vi "Pace pluse  interval Measurement.vi"(0 "ref in":T4, 1 "测试 类型":string(combo)="VREF", 5 "tasks in":T3, 7 "Oscilloscope IO":refnum<visa-resource-name>="tcpip0::192.168.40.220::instr", 9 "Data in":variant, 11 "error in (no error)":errorcluster) -> (6 "all  data out":T2={"conditions"={"do test?"=TRUE, "test name"="ib trim test", "user test name"="", "temp"=25.0, "spec min 1"=0.0, "spec max 1"=31.0, "spec min 2"=0.0, "spec max 2"=0.0, "spec units"="dec", "type"=enum."absolute", "vin inital"=2.8, "dwell initial"=0.5, "start"=0.0, "stop"=31.0, "step"=1.0, "dwell"=0.2, "bat imp"=0.0, "lead imp"=0.0, "schamber"="a", "gain"=0.0, "spolarity"="t2r", "as"=0.0, "vs"=0.0, "period"=0.0, "pchamber"="a", "ppolarity"="bip\nbip", "aamp"=0.0, "vamp"=0.0, "rchtime"=0.0, "rate"=0.0, "freq"=0.0, "vin end"=0.0, "dwell end"=0.5, "level a"=0.0, "level b"=0.0, "level c"=0.0, "level d"=0.0, "notes"="", "slew time"=25.0, "pw"=0.0, "times"=0.0, "spec min 3"=0.0, "spec max 3"=31.0, "spec min 4"=0.0, "spec max 4"=0.0}, "data out"=[], "result"=[], "TestArrayIndex"=0, "Result Measurement Head"=[]} {"conditions"."spec max 4" format="%^.3e"; "conditions"."spec min 4" format="%^.3e"; "conditions"."spec max 3" format="%^.3e"; "conditions"."spec min 3" format="%^.3e"; "conditions"."times" format="%^.3e"; "conditions"."pw" format="%^.3e"; "conditions"."slew time" format="%.2f"; "conditions"."level a" format="%^.3e"; "conditions"."freq" format="%^.3e"; "conditions"."rate" format="%^.3e"; "conditions"."rchtime" format="%^.3e"; "conditions"."vamp" format="%^.3e"; "conditions"."aamp" format="%^.3e"; "conditions"."period" format="%^.3e"; "conditions"."vs" format="%^.3e"; "conditions"."as" format="%^.3e"; "conditions"."gain" format="%^.3e"; "conditions"."lead imp" format="%^.3e"; "conditions"."bat imp" format="%^.3e"; "conditions"."spec max 2" format="%^.3e"; "conditions"."spec min 2" format="%^.3e"; "conditions"."level d" format="%^.3e"; "conditions"."level c" format="%^.3e"; "conditions"."level b" format="%^.3e"; "conditions"."dwell end" format="%^.3e"; "conditions"."vin end" format="%^.3e"; "conditions"."dwell" format="%^.3e"; "conditions"."step" format="%^.3e"; "conditions"."stop" format="%^.3e"; "conditions"."start" format="%^.3e"; "conditions"."dwell initial" format="%^.3e"; "conditions"."vin inital" format="%^.3e"; "conditions"."spec max 1" format="%^.3e"; "conditions"."spec min 1" format="%^.3e"; "conditions"."temp" format="%.2f"}, 10 "Measurement":string[](array[string]), 15 "Waveform Graph Cal":waveform(dbl)(graph))   [LabVIEW 2016]
uses:
  AET/TypeDef/Pacemaker ASIC Test_Reference.ctl
  AET/TypeDef/Pacemaker ASIC Test_Task.ctl
  AET/TypeDef/Pacemaker ASIC Test_Condition.ctl
  AET/TypeDef/Pacemaker ASIC Test_Register Mark Type.ctl
  Global Variables/Pacemaker ASIC Test_Save_SN Globals.vi
panel:
  out "Save_SN":path
  out "Pass/Fail":bool
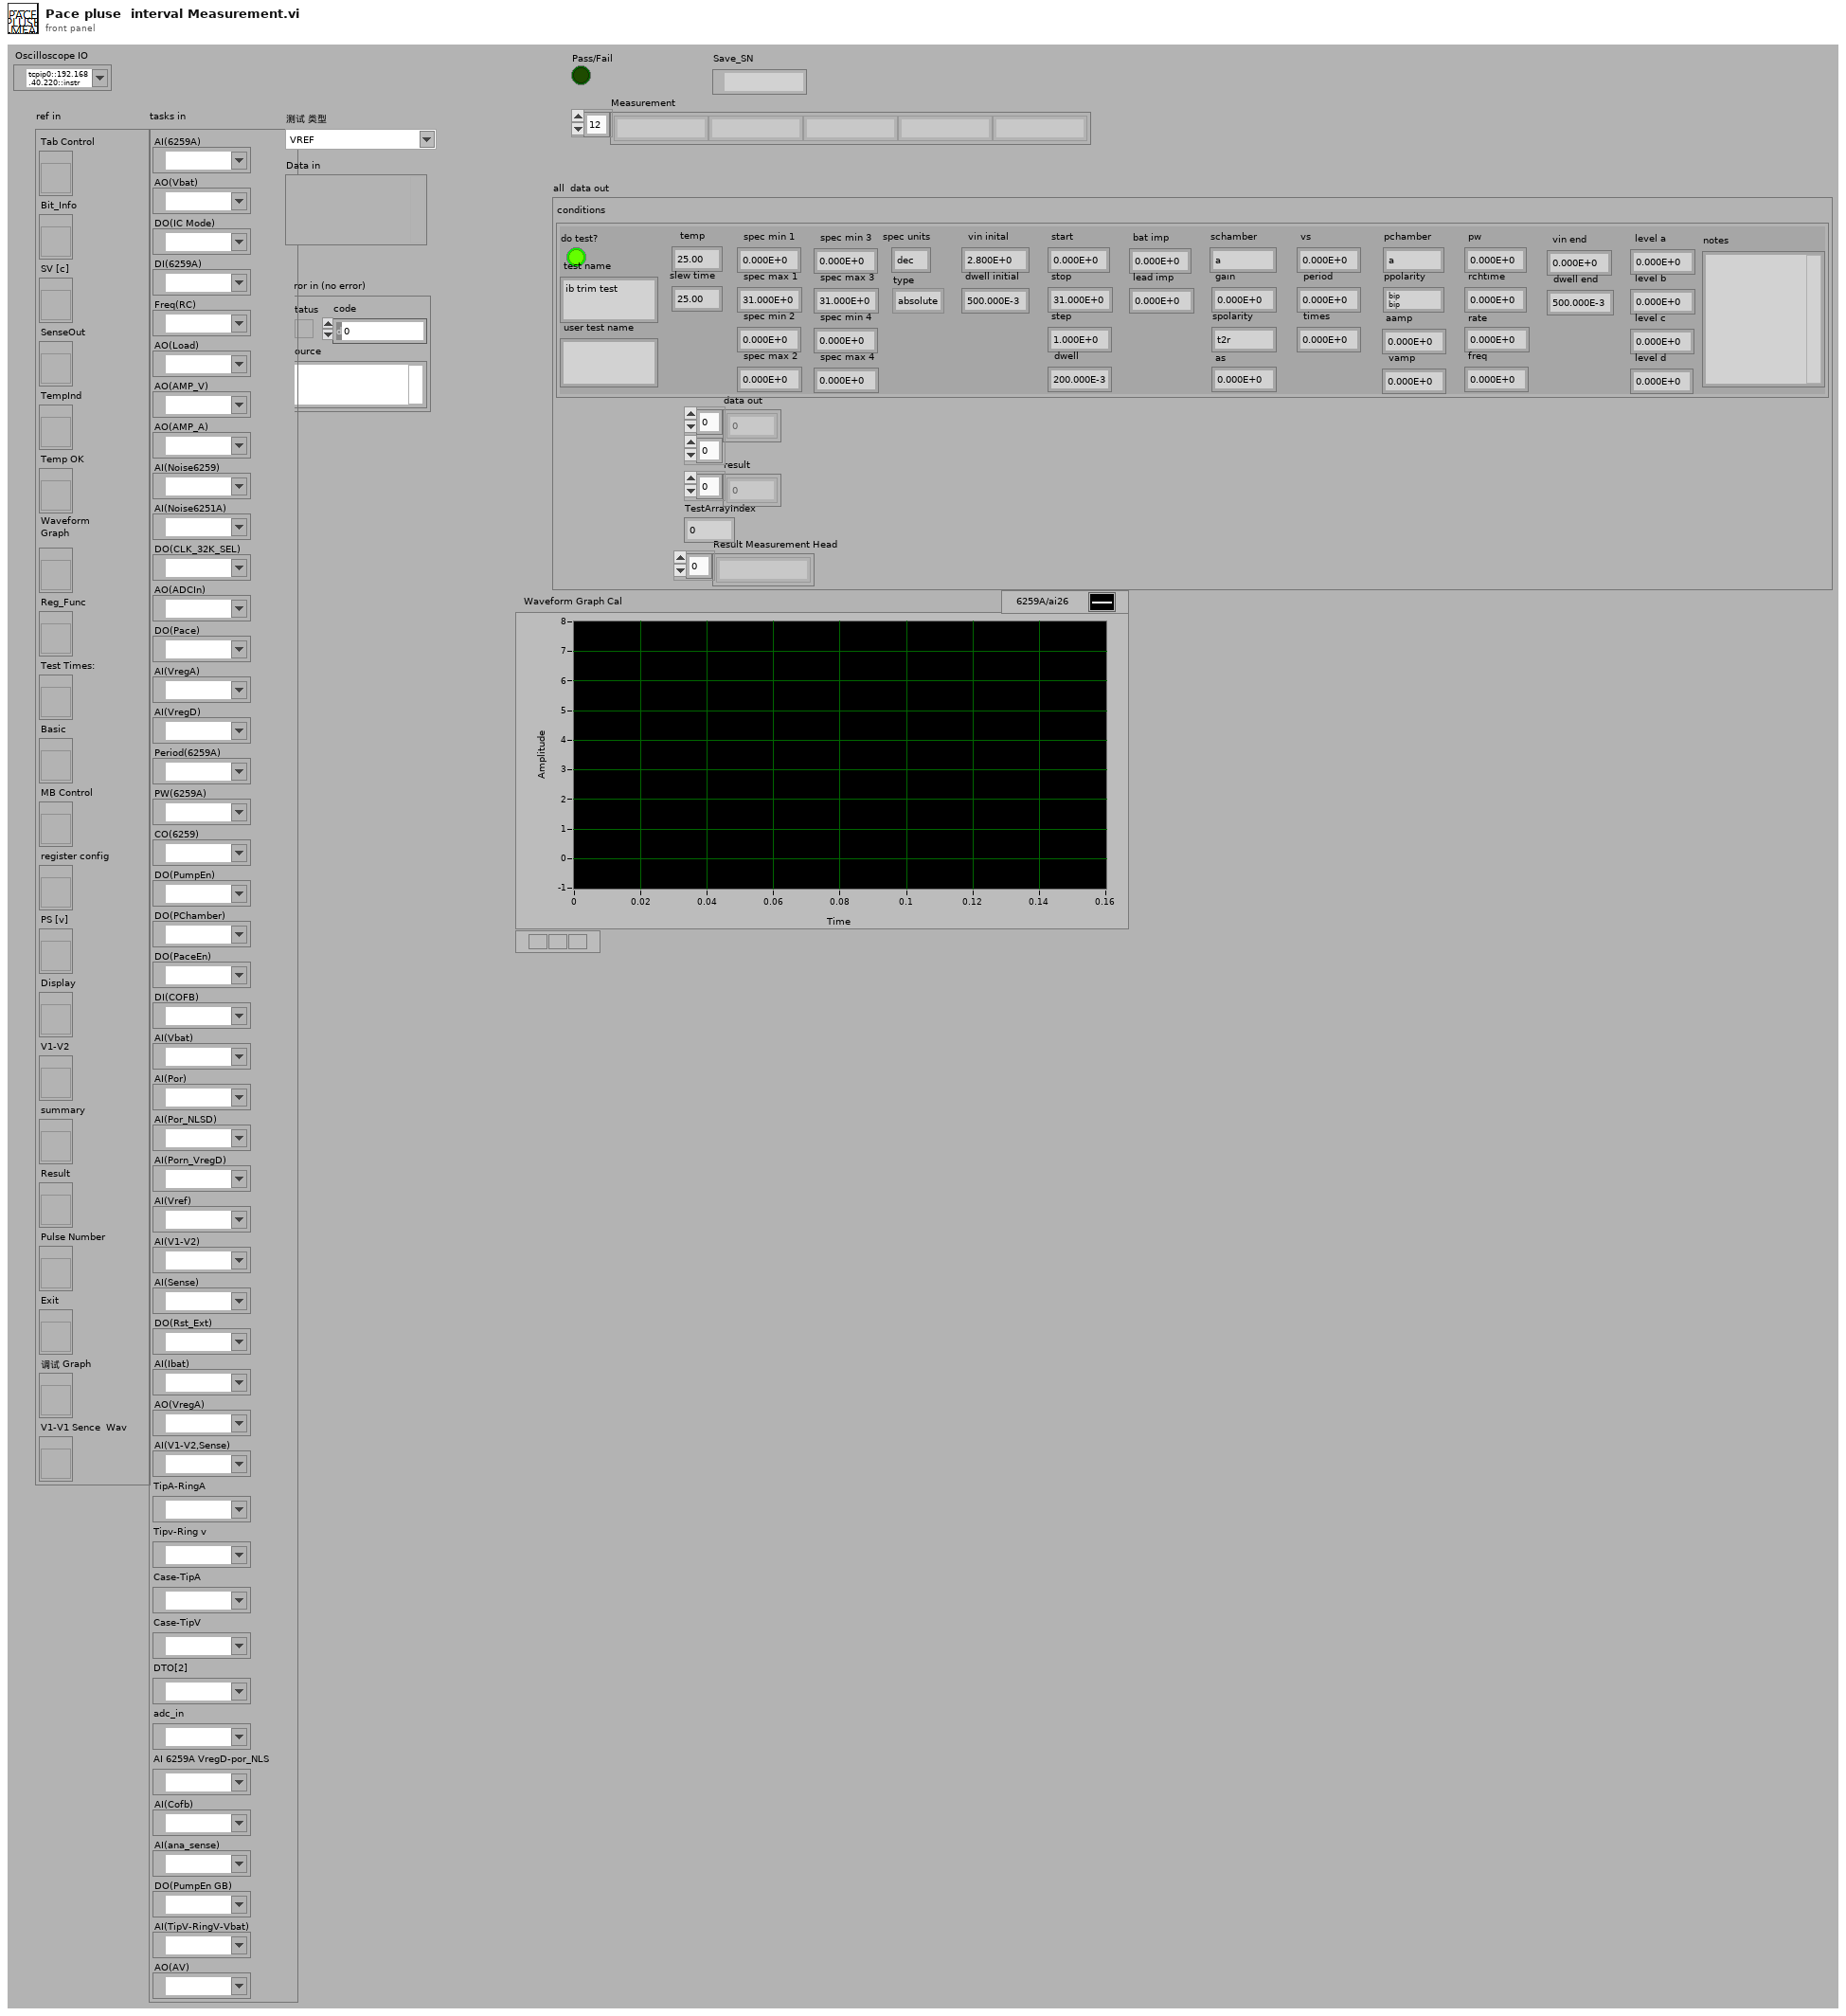
[diagram p1: front panel]
types:
  T1 = typedef "Pacemaker ASIC Test_Condition.ctl" = cluster{"do test?":bool, "test name":string, "user test name":string, "temp":dbl, "spec min 1":dbl, "spec max 1":dbl, "spec min 2":dbl, "spec max 2":dbl, "spec units":string, "type":enum16{"absolute", "v change", "pct change"}, "vin inital":dbl, "dwell initial":dbl, "start":dbl, "stop":dbl, "step":dbl, "dwell":dbl, "bat imp":dbl, "lead imp":dbl, "schamber":string, "gain":dbl, "spolarity":string, "as":dbl, "vs":dbl, "period":dbl, "pchamber":string, "ppolarity":string, "aamp":dbl, "vamp":dbl, "rchtime":dbl, "rate":dbl, "freq":dbl, "vin end":dbl, "dwell end":dbl, "level a":dbl, "level b":dbl, "level c":dbl, "level d":dbl, "notes":string, "slew time":dbl, "pw":dbl, "times":dbl, "spec min 3":dbl, "spec max 3":dbl, "spec min 4":dbl, "spec max 4":dbl}
  T2 = cluster{"conditions":T1, "data out":dbl[][], "result":dbl[], "TestArrayIndex":i32, "Result Measurement Head":string[]}
  T3 = typedef "Pacemaker ASIC Test_Task.ctl" = cluster{"AI(6259A)":refnum<k21>, "AO(Vbat)":refnum<k21>, "DO(IC Mode)":refnum<k21>, "DI(6259A)":refnum<k21>, "Freq(RC)":refnum<k21>, "AO(Load)":refnum<k21>, "AO(AMP_V)":refnum<k21>, "AO(AMP_A)":refnum<k21>, "AI(Noise6259)":refnum<k21>, "AI(Noise6251A)":refnum<k21>, "DO(CLK_32K_SEL)":refnum<k21>, "AO(ADCIn)":refnum<k21>, "DO(Pace)":refnum<k21>, "AI(VregA)":refnum<k21>, "AI(VregD)":refnum<k21>, "Period(6259A)":refnum<k21>, "PW(6259A)":refnum<k21>, "CO(6259)":refnum<k21>, "DO(PumpEn)":refnum<k21>, "DO(PChamber)":refnum<k21>, "DO(PaceEn)":refnum<k21>, "DI(COFB)":refnum<k21>, "AI(Vbat)":refnum<k21>, "AI(Por)":refnum<k21>, "AI(Por_NLSD)":refnum<k21>, "AI(Porn_VregD)":refnum<k21>, "AI(Vref)":refnum<k21>, "AI(V1-V2)":refnum<k21>, "AI(Sense)":refnum<k21>, "DO(Rst_Ext)":refnum<k21>, "AI(Ibat)":refnum<k21>, "AO(VregA)":refnum<k21>, "AI(V1-V2,Sense)":refnum<k21>, " TipA-RingA":refnum<k21>, "Tipv-Ring v":refnum<k21>, " Case-TipA":refnum<k21>, "Case-TipV":refnum<k21>, "DTO[2]":refnum<k21>, "adc_in":refnum<k21>, "AI 6259A VregD-por_NLS":refnum<k21>, "AI(Cofb)":refnum<k21>, "AI(ana_sense)":refnum<k21>, "DO(PumpEn GB)":refnum<k21>, "AI(TipV-RingV-Vbat)":refnum<k21>, "AO(AV)":refnum<k21>}
  T4 = typedef "Pacemaker ASIC Test_Reference.ctl" = cluster{"Tab Control":refnum<vi>, "Bit_Info":refnum<vi>, "SV [c]":refnum<vi>, "SenseOut":refnum<vi>, "TempInd":refnum<vi>, "Temp OK":refnum<vi>, "Waveform \nGraph":refnum<vi>, "Reg_Func":refnum<vi>, "Test Times:":refnum<vi>, "Basic":refnum<vi>, "MB Control":refnum<vi>, "register config":refnum<vi>, "PS [v]":refnum<vi>, "Display":refnum<vi>, "V1-V2":refnum<vi>, "summary":refnum<vi>, "Result":refnum<vi>, "Pulse Number":refnum<vi>, "Exit":refnum<vi>, "调试 Graph":refnum<vi>, "V1-V1 Sence  Wav ":refnum<vi>}
  T5 = typedef "Pacemaker ASIC Test_Register Mark Type.ctl" = enum16{"no action", "TRIM_BANDGAPV", "TRIM_VREGD", "TRIM_VREGA", "TRIM_IBIAS", "TRIM_HPFBW", "TRIM_LPFBW", "TRIM_RC32k", "TRIM_RC1p6k", "TRIM_IBIPT_A", "TRIM_IBIPT_V", "ASGN", "AS", "AUR_UT", "APAMP", "APW", "APUMPGN", "ARCHG", "ABILUNISEL", "VSGN", "VS", "VUR_UT", "VPAMP", "VPW", "VPUMPGN", "VRCHG", "VBILUNISEL", "Test_sel_a", "Test_sel_b", "DTO_SEL", "FBCMEN", "CPEN", "RC1p6kEN", "AntDTM", "ANTENN", "EGMFS REQ", "RC32kEN", "CPUOK", "ENOBLP1", "ENOBLP2", "OBLANK", "PDSA1", "PDSV1", "CSAEN", "CSVEN", "BIR RL", "BIR RH", "MREQ", "RK_SEL", "MRESULT1", "MRESULT2", "TrimOTA_0S1", "TrimOTA_0S2", "TrimOTV_0S1", "TrimOTV_0S2", "ENCASES", "TRIM_HPFBW_H_A", "TRIM_HPFBW_L_A", "TRIM_LPFBW_A", "TRIM_HPFBW_H_V", "TRIM_HPFBW_L_V", "TRIM_LPFBW_V", "R_C_Sel", "PDCHG", "ASIC VVI"}
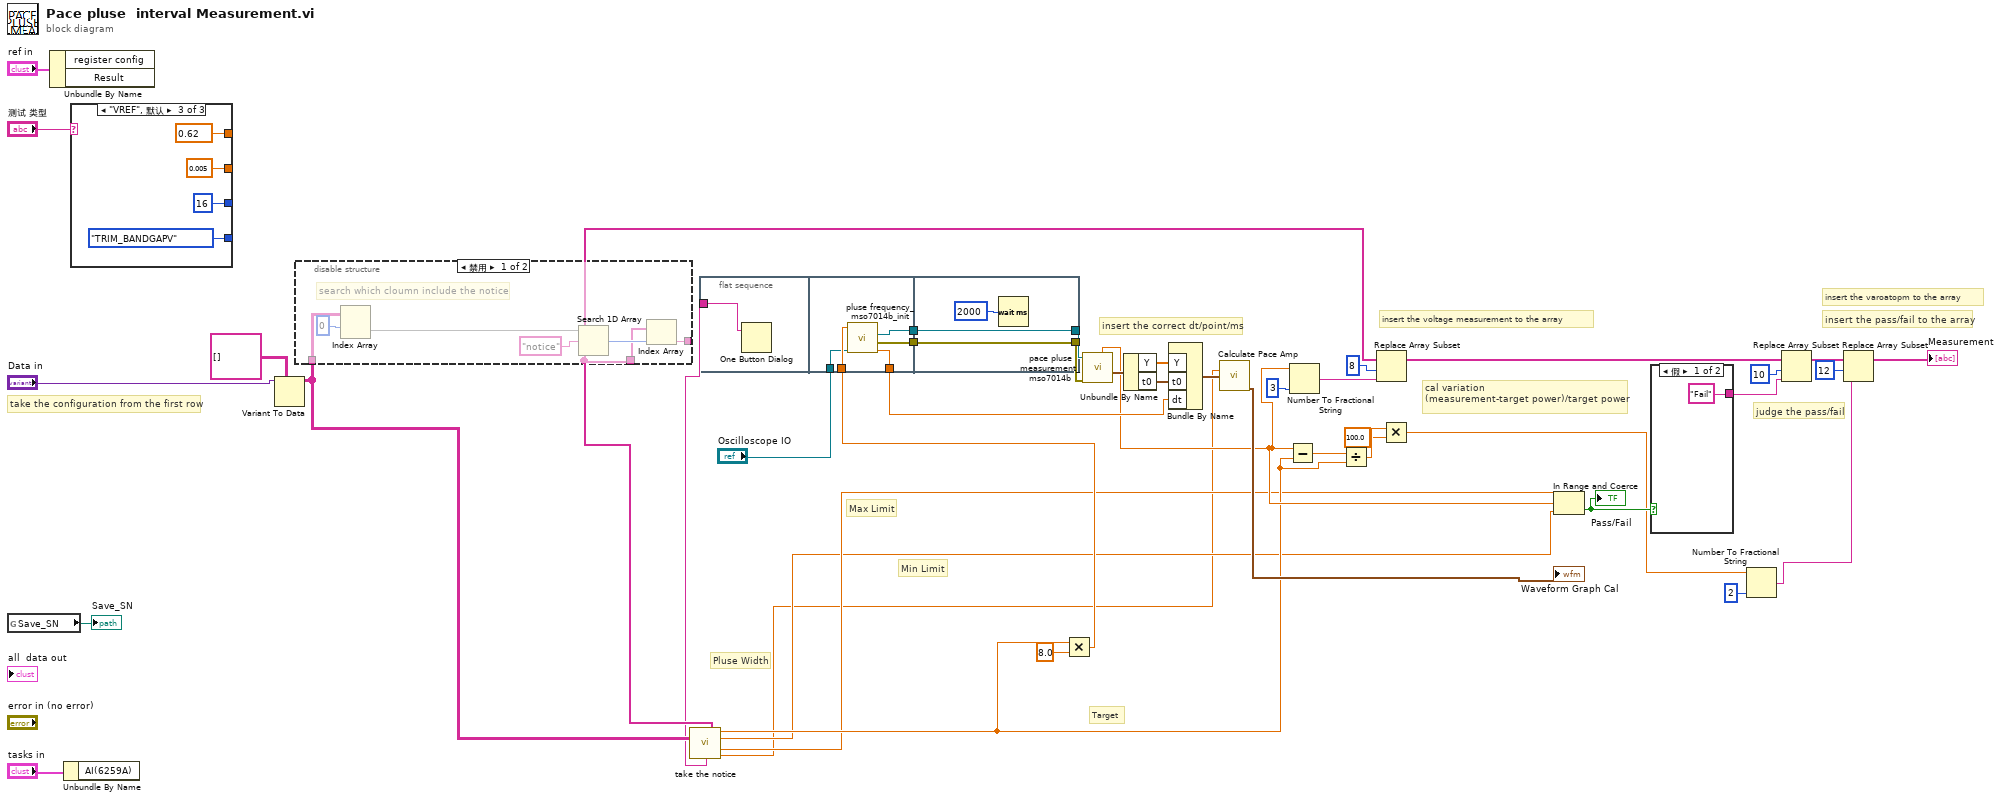
[diagram p0: block diagram]
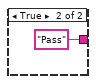
[diagram p3: hidden frame]
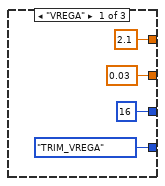
[diagram p4: hidden frame]
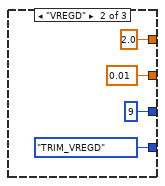
[diagram p5: hidden frame]
diagram:
  # "Pluse Width"
  # "insert the correct dt/point/ms"
  # "take the configuration from the first row"
  # "insert the pass/fail to the array"
  # "insert the varoatopm to the array"
  # "insert the voltage measurement to the array"
  # "judge the pass/fail"
  # "cal variation\n(measurement-target power)/target power"
  # "Target"
  # "Min Limit"
  # "Max Limit"
  n1 = global read "Pacemaker ASIC Test_Save_SN Globals.vi" "Save_SN"() -> (→"Save_SN":path)
  n2 = Unbundle By Name("ref in") -> ()  [unwired: 2 out]
  n3 = Unbundle By Name("tasks in") -> ()  [unwired: 1 out]
  n4 = case shown="\"VREF\", 默认" "测试 类型" {
    tunnel: [Pacemaker_ASIC_Test_Register_Mark_Type."TRIM_VREGA" ("Reg Mark") Pacemaker_ASIC_Test_Register_Mark_Type."TRIM_VREGD" ("Reg Mark") Pacemaker_ASIC_Test_Register_Mark_Type."TRIM_BANDGAPV" ("Reg Mark")] -> _
    tunnel: [2.1 ("y") 2.0 ("y") 0.62 ("y")] -> _
    tunnel: [u8 16 ("y") u8 9 ("y") u8 16 ("y")] -> _
    tunnel: [0.03 ("y") 0.01 ("y") 0.005 ("y")] -> _
    frame "VREGA" {
    }
    frame "VREGD" {
    }
    frame "VREF", Default {
    }
  }
  n5 = Variant To Data(type=string[][] [], Variant="Data in") -> (data=w8:string[][])  [unwired: 1 in, 1 out]
  n6 = call "take the notice.vi"("数组"=w8) -> ("Original array"=w3:string[], "Target"=w7:dbl, "Min"=w5:dbl, "Max"=w6:dbl, "notice"=w2:string, "Pluse Width"=w4:dbl)  [unwired: 7 in, 2 out]
  n7 = disable-structure shown="禁用" {
    disable-tunnel: [w58 _] -> _
    disable-tunnel: w3 -> [w57 _]
    disable-tunnel: w8 -> [w56 _]
    frame Disabled {
      # "search which cloumn include the notice"
      n8 = Index Array(array=w56, index (row)=0 ("索引 (行)")) -> (element=w61:string[])  [unwired: 1 in]
      n9 = Search 1D Array(1D array=w61, element="notice" ("元素")) -> (index of element=w59:i32)  [unwired: 1 in]
      n10 = Index Array(array=w57, index=w59) -> (element=w58:string)
    }
    frame Enabled {
    }
  }
  n11 = flat-sequence {
    tunnel: w2 -> [w63]
    tunnel: [w68] -> w33
    tunnel: [w67] -> w32
    tunnel: [w66] -> w25
    tunnel: w16 -> [w65]
    tunnel: "Oscilloscope IO" -> [w64]
    tunnel: [w70] -> w37
    tunnel: [w71] -> w38
    tunnel: w33 -> [w71]
    tunnel: w32 -> [w70]
    frame #0 {
      n12 = One Button Dialog(message=w63) -> ()  [unwired: 1 in, 1 out]
    }
    frame #1 {
      n13 = call "pluse frequency_mso7014b_init.vi"("VISA resource name"=w64, "Timebase (20.0E-9)"=w65) -> ("dt"=w66:dbl, "error out"=w67:errorcluster, "VISA resource name out"=w68:refnum<visa-resource-name>)  [unwired: 7 in]
    }
    frame #2 {
      n14 = Wait (ms)(milliseconds to wait=u32 2000 ("等待时间（毫秒）")) -> ()  [unwired: 1 out]
    }
  }
  n15 = Multiply(x=w7, y=8.0) -> (x*y=w16:dbl)
  n16 = call "pace pluse measurement_mso7014b.vi"("error in (no error)"=w37, "VISA resource name"=w38) -> ("CH1 Waveform"=w24:waveform(dbl), "Pluse Interval"=w9:dbl)  [unwired: 5 in, 3 out]
  n17 = Unbundle By Name(w24) -> ("Y"=w27:dbl[], "t0"=w26:timestamp)
  n18 = Bundle By Name("Y"=w27, "t0"=w26, "dt"=w25) -> (w23:waveform(dbl))  [unwired: 1 in]
  n19 = call "Calculate Pace Amp.vi"("设定脉宽"=w4, "Test Result"=w23) -> ("Waveform Graph Cal"=→"Waveform Graph Cal":waveform(dbl))  [unwired: 4 in, 9 out]
  n20 = Subtract(x=w9, y=w7) -> (x-y=w20:dbl)
  n21 = Number To Fractional String(number=w9, precision (6)=i16 3 ("精度(6)")) -> (F-format string=w35:string)  [unwired: 2 in]
  n22 = Divide(x=w20, y=w7) -> (x/y=w19:dbl)
  n23 = Replace Array Subset(array=w3, new element=w35, index=8 ("索引")) -> (w21:string[])
  n24 = Multiply(x=w19, y=100.0) -> (x*y=w14:dbl)
  n25 = In Range and Coerce(upper limit=w6, x=w9, lower limit=w5) -> (In Range?=w31:bool)  [unwired: 1 out]
  "Pass/Fail" <- w31
  n26 = case shown="假" w31 {
    tunnel: ["Fail" "Pass"] -> w30
    frame False {
    }
    frame True {
    }
  }
  n27 = Number To Fractional String(number=w14, precision (6)=i16 2 ("精度(6)")) -> (F-format string=w12:string)  [unwired: 2 in]
  n28 = Replace Array Subset(array=w21, new element=w30, index=10 ("索引")) -> (w15:string[])
  n29 = Replace Array Subset(array=w15, new element=w12, index=12 ("索引")) -> (→"Measurement":string[])
